vi "Make New Worker.vi"(8 "New Project?":bool, 9 "Add to Project (None)":refnum<vi>, 11 "New Worker Name":string) -> (0 "error out":errorcluster)   [LabVIEW 2020, in "FlexBlocks.lvlib"]
uses:
  FlexBlocks.lvlib
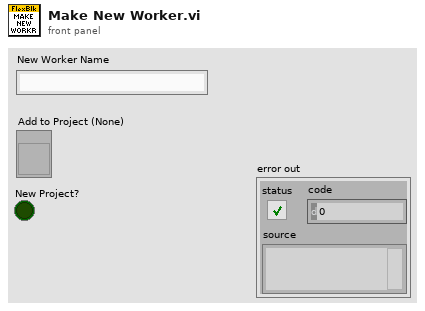
[diagram p1: front panel]
types:
  T1 = typedef "FlexBlocks.lvlib/Paths.ctl" = cluster{"FlexBlocks":path, "Workers Root":path, "Specialized Editors":path, "Worker Template":path, "Editor Template":path, "Express Template":path}
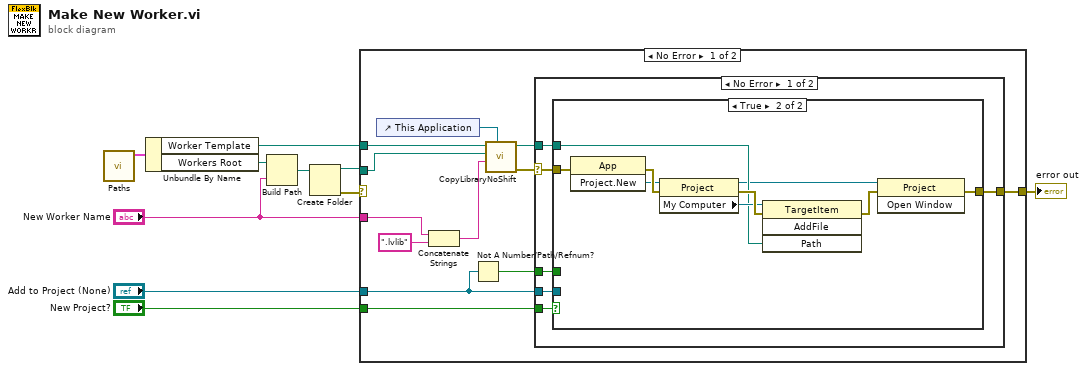
[diagram p0: block diagram]
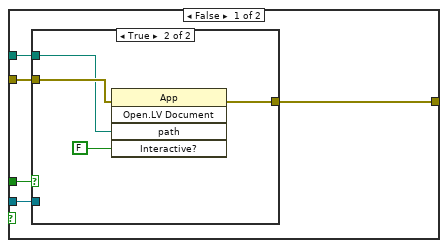
[diagram p2: hidden frame]
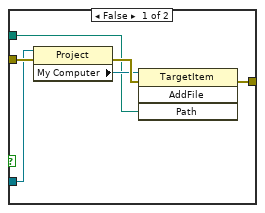
[diagram p3: hidden frame]
diagram:
  n1 = call "Paths.vi"() -> ("Paths"=w10:T1)  [unwired: 11 in]
  n2 = Unbundle By Name(w10) -> ("Worker Template"=w4:path, "Workers Root"=w9:path)
  n3 = Build Path(base path=w9, name or relative path="New Worker Name") -> (appended path=w8:path)
  n4 = Create Folder(path (use dialog)=w8) -> (created path=w6:path, error out=w7:errorcluster)  [unwired: 2 in, 1 out]
  n5 = case shown="No Error" w7 {
    selector: w7 -> [_ w54]
    tunnel: w6 -> [w16 _]
    tunnel: "New Worker Name" -> [w21 _]
    tunnel: w4 -> [w19 _]
    tunnel: [w14 w54] -> w3
    tunnel: "Add to Project (None)" -> [w12 _]
    tunnel: "New Project?" -> [w13 _]
    frame No Error {
      n6 = control-ref of="This Application"() -> (w18:refnum<vi>)
      n7 = Concatenate Strings(w21, ".lvlib" ("string")) -> (w17:string)
      n8 = Not A Number/Path/Refnum?(number/path/refnum=w12) -> (NaN/Path/Refnum?=w11:bool)
      n9 = call "CopyLibraryNoShift.vi"("app"=w18, "new library name"=w17, "new folder"=w16, "source library path"=w19) -> ("error out"=w22:errorcluster, "copied library path"=w15:path)  [unwired: 5 in, 1 out]
      n10 = case shown="No Error" w22 {
        selector: w22 -> [w28 w53]
        tunnel: w15 -> [w27 _]
        tunnel: [w26 w53] -> w14
        tunnel: w13 -> [w25 _]
        tunnel: w12 -> [w24 _]
        tunnel: w11 -> [w23 _]
        frame No Error {
          n11 = case shown="True" w25 {
            tunnel: w28 -> [w33 w47]
            tunnel: w27 -> [w32 w48]
            tunnel: [w31 w44] -> w26
            tunnel: w24 -> [w29 _]
            tunnel: w23 -> [w30 _]
            frame False {
              n12 = case shown="True" w30 {
                tunnel: w33 -> [w39 w43]
                tunnel: w32 -> [w35 w41]
                tunnel: [w34 w40] -> w31
                tunnel: w29 -> [w37 _]
                frame False {
                  n13 = property class="Project"(reference=w37, error in=w39) -> (error out=w38:errorcluster, "My Computer"=w36:refnum<vi>)  [unwired: 1 out]
                  n14 = invoke class="TargetItem" method="AddFile"(reference=w36, error in=w38, "Path"=w35) -> (error out=w34:errorcluster)  [unwired: 1 in, 3 out]
                }
                frame True {
                  n15 = invoke class="App" method="Open.LV Document"(error in=w43, "path"=w41, "Interactive?"=FALSE) -> (error out=w40:errorcluster)  [unwired: 2 in, 4 out]
                }
              }
            }
            frame True {
              n16 = invoke class="App" method="Project.New"(error in=w47) -> (error out=w51:errorcluster, "Project:New"=w50:refnum<vi>)  [unwired: 2 in, 1 out]
              n17 = property class="Project"(reference=w50, error in=w51) -> (reference out=w46:refnum<vi>, error out=w52:errorcluster, "My Computer"=w49:refnum<vi>)
              n18 = invoke class="TargetItem" method="AddFile"(reference=w49, error in=w52, "Path"=w48) -> (error out=w45:errorcluster)  [unwired: 1 in, 3 out]
              n19 = invoke class="Project" method="Open Window"(reference=w46, error in=w45) -> (error out=w44:errorcluster)  [unwired: 1 in, 2 out]
            }
          }
        }
        frame Error {
        }
      }
    }
    frame Error {
    }
  }
  "error out" <- w3
